vi "measure.vi"(8 "error in (no error)":errorcluster, 11 "connection ID":refnum<k5>) -> (0 "error out":errorcluster, 2 "Temperature (C)":dbl, 3 "connection ID out":refnum<k5>)   [LabVIEW 2018]
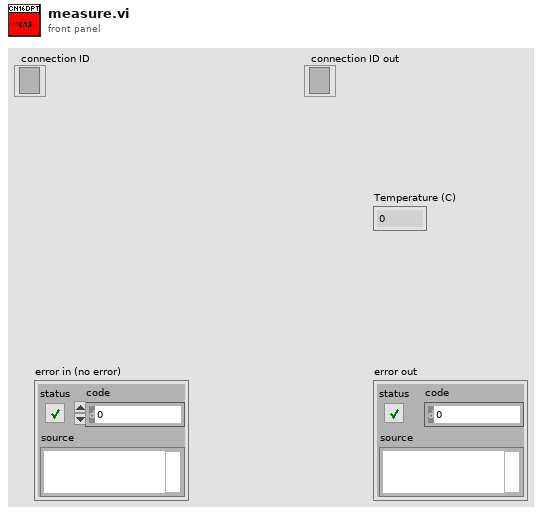
[diagram p1: front panel]
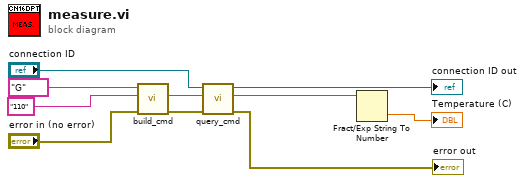
[diagram p0: block diagram]
diagram:
  n1 = call "build_cmd.vi"("error in (no error)"="error in (no error)", "Command ID"="110", "Command class"="G") -> ("error out"=w7:errorcluster, "Command"=w6:string)  [unwired: 7 in]
  n2 = call "query_cmd.vi"("error in (no error)"=w7, "Command"=w6, "connection ID"="connection ID") -> ("error out"=→"error out":errorcluster, "Response"=w5:string, "connection ID out"=→"connection ID out":refnum<k5>)  [unwired: 6 in]
  n3 = Fract/Exp String To Number(string=w5) -> (number=→"Temperature (C)":dbl)  [unwired: 3 in, 1 out]
